vi "Initialize EtherCAT Output Frame.vi"(1 "Bus Setup":T2) -> (0 "EtherCAT Output Frame":T1 format="%.0x")   [LabVIEW 2024, in "EtherCAT Model.lvlib"]
uses:
  EtherCAT Model.lvlib
  <instrlib>/_Ackermann Automation/EtherCAT Lib/EcatLib/TypeDefs/ClusterBusSetup.ctl
  <instrlib>/_Ackermann Automation/EtherCAT Lib/EcatLib/EthercatLib.lvlib
  EtherCAT Output Data Frame.ctl
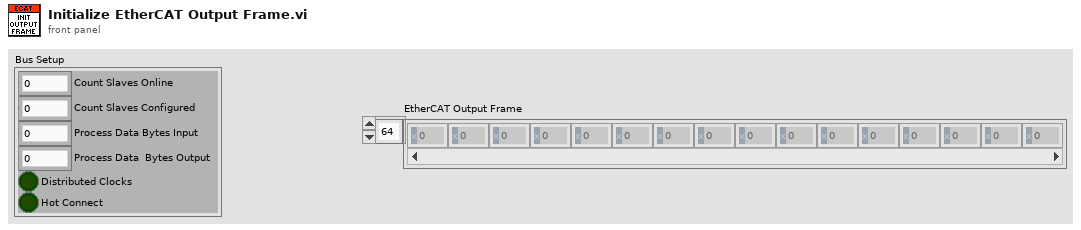
[diagram p1: front panel]
types:
  T1 = typedef "EtherCAT Model.lvlib/EtherCAT Output Data Frame.ctl" = u8[]
  T2 = typedef "EthercatLib.lvlib/ClusterBusSetup.ctl" = cluster{"Count Slaves Online":u32, "Count Slaves Configured":u32, "Process Data Bytes Input":u32, "Process Data  Bytes Output":u32, "Distributed Clocks":bool, "Hot Connect":bool}
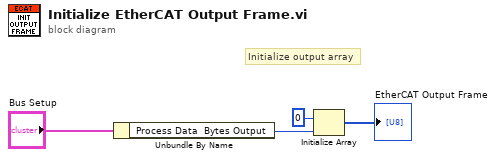
[diagram p0: block diagram]
diagram:
  # "Initialize output array"
  n1 = Unbundle By Name("Bus Setup") -> ("Process Data  Bytes Output"=w4:u32)
  n2 = Initialize Array(u8 0, w4) -> (→"EtherCAT Output Frame":u8[])
